vi "readBaseILCSettings.vi"(8 "error in (no error)":errorcluster, 11 "Boot in":refnum<class "Boot.lvclass">) -> (0 "error out":errorcluster, 2 "BaseHardpointSettings":T1, 3 "Boot out":refnum<class "Boot.lvclass">)   [LabVIEW 2016, in "Boot.lvclass"]
uses:
  Boot.lvclass
  DataTypes/Settings/Base/BaseILCSettings.ctl
  Common_RT_ILC/DataTypes/ILCTimings.ctl
  Boot.lvclass/Boot.ctl
  Settings/Settings/Setting.lvclass
  Common_RT_ILC/RTILC.lvlib
  DataTypes/Settings/M1M3SupportSettings.lvlib
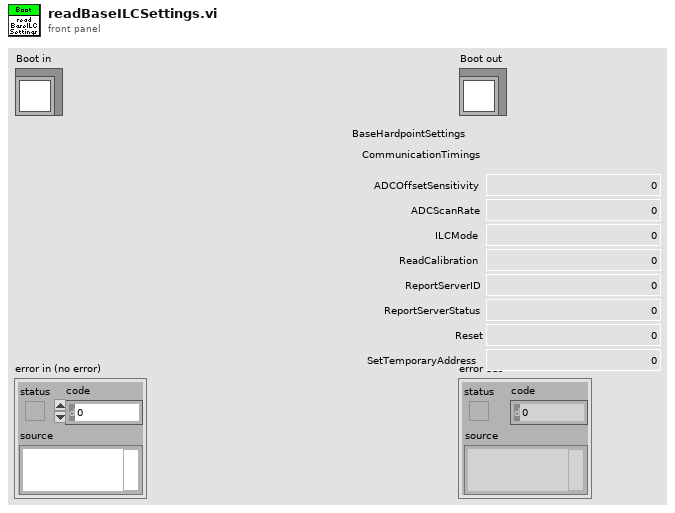
[diagram p1: front panel]
types:
  T1 = typedef "M1M3SupportSettings.lvlib/BaseILCSettings.ctl" = cluster{"CommunicationTimings":T2}
  T2 = typedef "RTILC.lvlib/ILCTimings.ctl" = cluster{"ADCOffsetSensitivity":u32, "ADCScanRate":u32, "ILCMode":u32, "ReadCalibration":u32, "ReportServerID":u32, "ReportServerStatus":u32, "Reset":u32, "SetTemporaryAddress":u32}
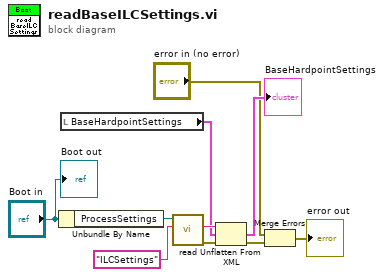
[diagram p0: block diagram]
diagram:
  n1 = Unbundle By Name("Boot in") -> ("ProcessSettings"=w10:refnum<class "Setting.lvclass">)
  n2 = local read "BaseHardpointSettings"() -> (w7:T1)
  n3 = call-dynamic "read.vi"("Name"="ILCSettings", "BaseSetting in"=w10) -> ("error out"=w4:errorcluster, "XML"=w8:string)  [unwired: 6 in, 2 out]
  n4 = Unflatten From XML(xml string=w8, type=w7, error in (no error)=w4) -> (value=→"BaseHardpointSettings":T1, error out=w1:errorcluster)
  n5 = Merge Errors("error in (no error)", w1) -> (→"error out":errorcluster)
  "Boot out" <- "Boot in"
